vi "Configure Fold.vi"(8 "error in (no error)":errorcluster, 10 "Fold Setting (0, OFF)":u16(ring) items=["OFF", "CV", "CC"], 11 "VISA resource name":refnum<visa-resource-name>) -> (0 "error out":errorcluster, 3 "VISA resource name out":refnum<visa-resource-name>)   [LabVIEW 2021, in "Sorensen M9A Series.lvlib"]
doc: "This VI sets the Sorensen power supply's foldback mode, which disables output when the foldback condition is entered. Can be set to 0 (off), 1 (constant voltage), or 2 (constant current)."
uses:
  Sorensen M9A Series.lvlib
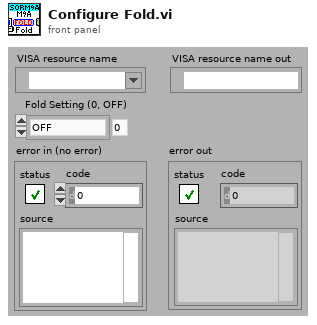
[diagram p1: front panel]
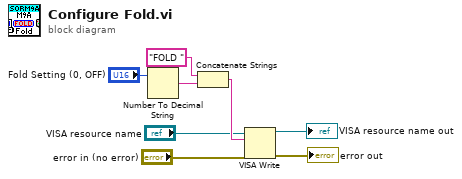
[diagram p0: block diagram]
diagram:
  n1 = Number To Decimal String(number="Fold Setting (0, OFF)") -> (decimal integer string=w3:string)  [unwired: 1 in]
  n2 = Concatenate Strings("FOLD ", w3) -> (w5:string)
  n3 = VISA Write(VISA resource name="VISA resource name", write buffer=w5, error in (no error)="error in (no error)") -> (VISA resource name out=→"VISA resource name out":refnum<visa-resource-name>, error out=→"error out":errorcluster)  [unwired: 1 out]
